vi "Map data rate.vi"(11 "Data Rate In":string) -> (3 "Data Rate Out":string)   [LabVIEW 2011]
panel:
  in  "Data Rate":string(combo)="1,0,0"
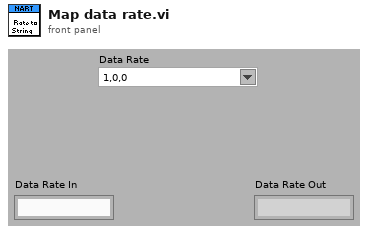
[diagram p1: front panel]
types:
  T1 = typedef "LVComboBoxStrsAndValuesArrayTypeDef.ctl" = cluster{"String":string, "Value":string}[]
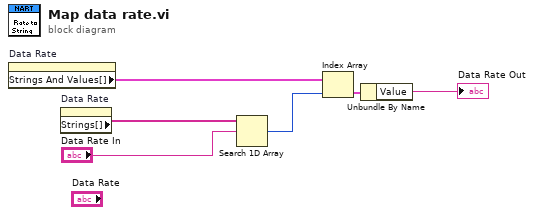
[diagram p0: block diagram]
diagram:
  n1 = property on="Data Rate" class="CmbBox"() -> ("Strings And Values[]"=w4:T1)  [unwired: 2 in, 2 out]
  n2 = property on="Data Rate" class="CmbBox"() -> ("Strings[]"=w5:string[])  [unwired: 2 in, 2 out]
  n3 = Search 1D Array(1D array=w5, element="Data Rate In") -> (index of element=w2:i32)  [unwired: 1 in]
  n4 = Index Array(array=w4, index=w2) -> (element=w1:cluster{"String":string, "Value":string})
  n5 = Unbundle By Name(w1) -> ("Value"=→"Data Rate Out":string)
